vi "Handle LogRec.vi"(8 "error in":errorcluster, 10 "LogRecord":refnum<class "LogRecord.lvclass">, 11 "FileHandler in":refnum<class "FileHandler.lvclass">) -> (0 "error out":errorcluster, 3 "FileHandler out":refnum<class "FileHandler.lvclass">)   [LabVIEW 2020, in "hse-logger.lvlib" / "FileHandler.lvclass"]
doc: "Handles the incoming ``LogRecord`` object. If the level of the record is greater or equal to the level of the handler, then the record is written to the file. \n\n____\nHAMPEL SOFTWARE ENGINEERING v2.0.6 (2021-04-15 11:38)"
uses:
  FileHandler.lvclass
  LogRecord/LogRecord.lvclass
  LogRecord/LogRecord.lvclass/LogRecord.ctl
  FileHandler.lvclass/FileHandler.ctl
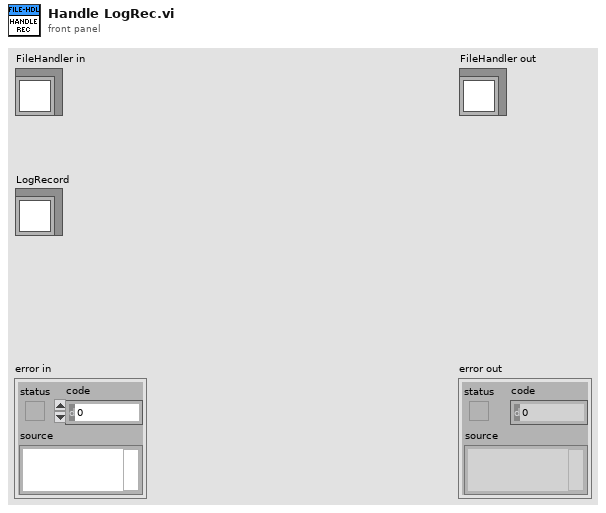
[diagram p1: front panel]
types:
  T1 = typedef "hse-logger.lvlib/LogLevel.ctl" = enum16{"DEBUG", "INFO", "WARNING", "ERROR", "CRITICAL"}
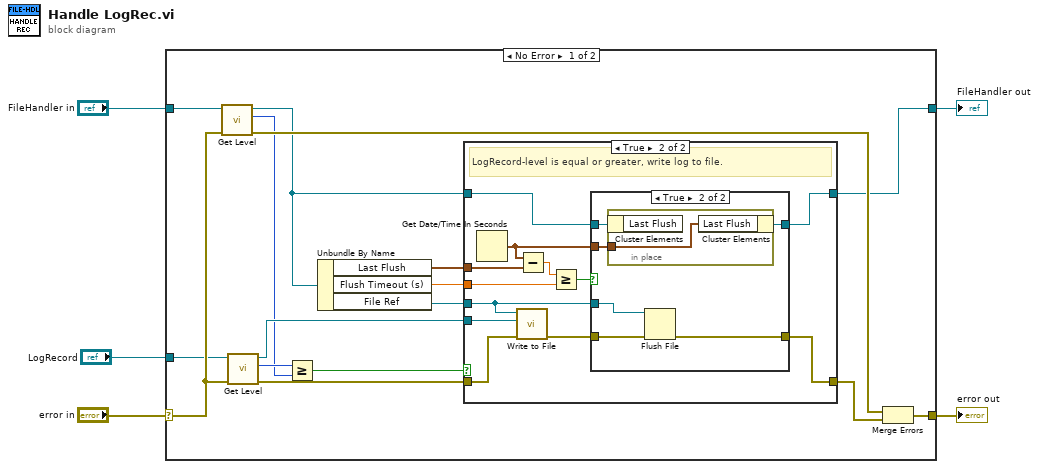
[diagram p0: block diagram]
diagram:
  n1 = case shown="No Error" "error in" {
    selector: "error in" -> [w20 w46]
    tunnel: [w10 w46] -> w4
    tunnel: [w6 w45] -> w2
    tunnel: "FileHandler in" -> [w17 w45]
    tunnel: "LogRecord" -> [w19 _]
    frame No Error {
      n2 = call-dynamic "Get Level.vi"("error in"=w20, "Handler in"=w17) -> ("error out"=w21:errorcluster, "Level"=w15:T1, "Handler out"=w7:refnum<class "FileHandler.lvclass">)  [unwired: 7 in]
      n3 = call "Get Level.vi"("error in"=w20, "LogRecord in"=w19) -> ("error out"=w13:errorcluster, "Level"=w16:T1, "LogRecord out"=w18:refnum<class "LogRecord.lvclass">)  [unwired: 7 in]
      n4 = Greater Or Equal?(x=w16, y=w15) -> (x >= y?=w14:bool)
      n5 = Unbundle By Name(w7) -> ("Last Flush"=w9:timestamp, "Flush Timeout (s)"=w8:dbl, "File Ref"=w12:refnum<file>)
      n6 = case shown="True" w14 {
        tunnel: w18 -> [_ w35]
        tunnel: w13 -> [w23 w34]
        tunnel: w12 -> [_ w28]
        tunnel: [w23 w25] -> w11
        tunnel: w9 -> [_ w33]
        tunnel: w8 -> [_ w31]
        tunnel: w7 -> [w22 w26]
        tunnel: [w22 w24] -> w6
        frame False {
          # "Do not write to file."
        }
        frame True {
          # "LogRecord-level is equal or greater, write log to file."
          n7 = Get Date/Time In Seconds() -> (seconds since 1Jan1904=w27:timestamp)
          n8 = call "Write to File.vi"("error in"=w34, "LogRecord in"=w35, "File Ref"=w28) -> ("error out"=w29:errorcluster)  [unwired: 8 in]
          n9 = Subtract(x=w27, y=w33) -> (x-y=w32:dbl)
          n10 = Greater Or Equal?(x=w32, y=w31) -> (x >= y?=w30:bool)
          n11 = case shown="True" w30 {
            tunnel: w29 -> [w36 w43]
            tunnel: w28 -> [_ w42]
            tunnel: w27 -> [_ w38]
            tunnel: w26 -> [w37 w40]
            tunnel: [w37 w39] -> w24
            tunnel: [w36 w41] -> w25
            frame False {
            }
            frame True {
              n12 = in-place {
                in-place-border: w38 -> [w44]
                n13 = in-place-cluster #1(w40) -> ()  [unwired: 1 out]
                n14 = in-place-cluster #1("Last Flush"=w44) -> (w39:refnum<class "FileHandler.lvclass">)
              }
              n15 = Flush File(refnum=w42, error in=w43) -> (error out=w41:errorcluster)  [unwired: 1 out]
            }
          }
        }
      }
      n16 = Merge Errors(w21, w11) -> (w10:errorcluster)
    }
    frame Error {
    }
  }
  "error out" <- w4
  "FileHandler out" <- w2
